vi "lxw parse cols.vi"(8 "error in (no error)":errorcluster, 9 "last_col":u16, 10 "first_col":u16, 11 "cols_str":string) -> (0 "error out":errorcluster, 1 "last_col out":u16, 2 "first_col out":u16)   [LabVIEW 2015, in "xlsxwriter.lvlib"]
doc: "void lxw_parse_cols(const char *cols_str, lxw_col_t *first_col, lxw_col_t *last_col);"
uses:
  xlsxwriter.lvlib
  xlsxwriter.dll
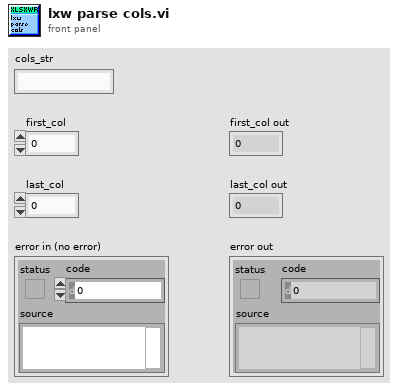
[diagram p1: front panel]
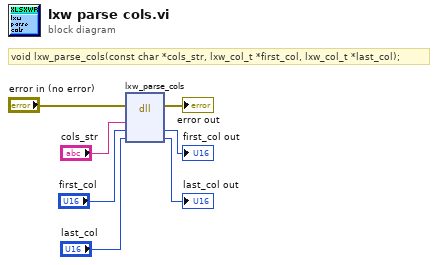
[diagram p0: block diagram]
diagram:
  # "void lxw_parse_cols(const char *cols_str, lxw_col_t *first_col, lxw_col_t *last_col);"
  n1 = dll-call lib="C:/Users/WDAGUtilityAccount/Desktop/lv_vis_added_cell/xlsxwriter.*" fn="lxw_parse_cols"(error in="error in (no error)", "cols_str"="cols_str", "first_col"="first_col", "last_col"="last_col") -> (error out=→"error out":errorcluster, "first_col"=→"first_col out":u16, "last_col"=→"last_col out":u16)  [unwired: 4 in, 1 out]
